vi "Calculate Intersection.vi"(8 "Dy":dbl[](array[numeric]), 9 "Dx":dbl[](array[numeric]), 10 "Cy":dbl[](array[numeric]), 11 "Cx":dbl[](array[numeric])) -> (0 "Found?":bool, 2 "Y":dbl[](array[numeric]), 3 "X":dbl[](array[numeric]))   [LabVIEW 2023, in "d15.lvlib" / "Cave.lvclass"]
uses:
  Cave.lvclass
  <vilib>/Analysis/NI_AAL_Geometry.lvlib
  Diamond/Diamond.lvclass
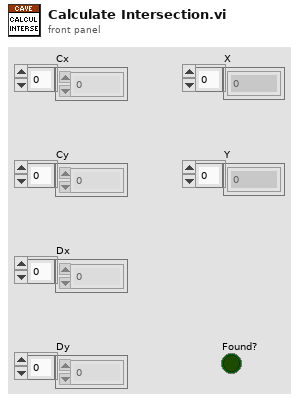
[diagram p1: front panel]
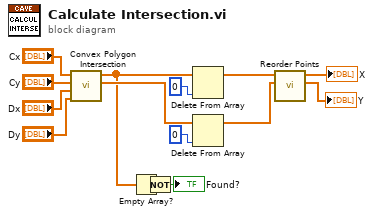
[diagram p0: block diagram]
diagram:
  n1 = call <vilib>:"Convex Polygon Intersection.vi"("Y 2"="Dy", "X 2"="Dx", "Y 1"="Cy", "X 1"="Cx") -> ("Intersection Y"=w14:dbl[], "Intersection X"=w3:dbl[])  [unwired: 5 in, 1 out]
  n2 = Empty Array?(array=w3) -> (empty?=w2:bool)
  n3 = Not(x=w2) -> (.not. x?=→"Found?":bool)
  n4 = Delete From Array(array=w3, index=0) -> (array with subset deleted=w7:dbl[])  [unwired: 1 in, 1 out]
  n5 = Delete From Array(array=w14, index=0) -> (array with subset deleted=w6:dbl[])  [unwired: 1 in, 1 out]
  n6 = call "Reorder Points.vi"("Y"=w6, "X"=w7) -> ("Y'"=→"Y":dbl[], "X'"=→"X":dbl[])  [unwired: 8 in]
